vi "Shot Counter.vi"() -> ()   [LabVIEW 2013]
uses:
  <vilib>/Utility/file.llb/Write To Spreadsheet File (DBL).vi
  <vilib>/Utility/file.llb/Read From Spreadsheet File (I64).vi
  <vilib>/Utility/file.llb/Write To Spreadsheet File (I64).vi
  Globals/Useful Values.vi
panel:
  out "Time":i64
  out "Shots":i64
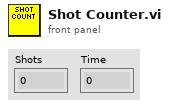
[diagram p1: front panel]
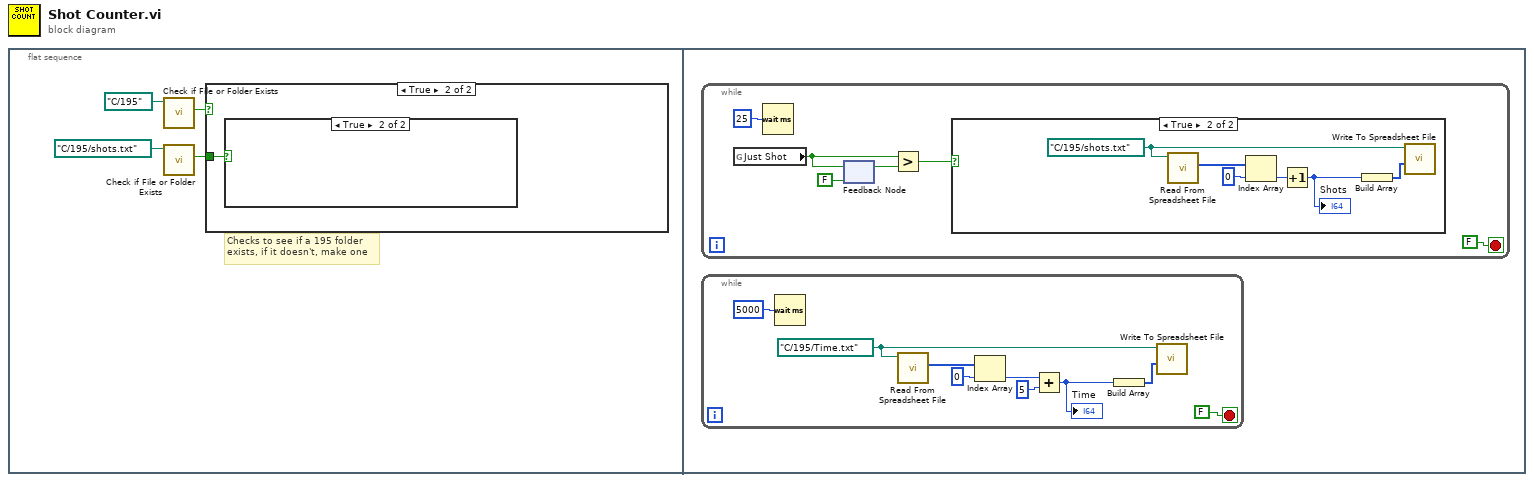
[diagram p0: block diagram]
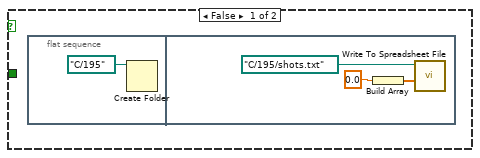
[diagram p2: hidden frame]
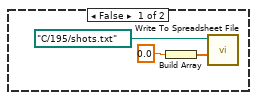
[diagram p3: hidden frame]
diagram:
  n1 = flat-sequence {
    frame #0 {
      # "Checks to see if a 195 folder\nexists, if it doesn't, make one"
      n2 = call <vilib>:"Check if File or Folder Exists.vi"("path"=path "C:/195") -> ("file or folder exists?"=w2:bool)  [unwired: 8 in, 2 out]
      n3 = call <vilib>:"Check if File or Folder Exists.vi"("path"=path "C:/195/shots.txt") -> ("file or folder exists?"=w1:bool)  [unwired: 8 in, 2 out]
      n4 = case shown="True" w2 {
        tunnel: w1 -> [_ w9]
        frame False {
          n5 = flat-sequence {
            frame #0 {
              n6 = Create Folder(path (use dialog)=path "C:/195") -> ()  [unwired: 2 in, 3 out]
            }
            frame #1 {
              n7 = Build Array(0.0 ("element")) -> (w7:dbl[])
              n8 = call-poly <vilib>:"Write To Spreadsheet File.vi"("1D data"=w7, "file path (dialog if empty)"=path "C:/195/shots.txt") -> ()  [unwired: 6 in, 1 out]
            }
          }
        }
        frame True {
          n9 = case shown="True" w9 {
            frame False {
              n10 = Build Array(0.0 ("element")) -> (w11:dbl[])
              n11 = call-poly <vilib>:"Write To Spreadsheet File.vi"("1D data"=w11, "file path (dialog if empty)"=path "C:/195/shots.txt") -> ()  [unwired: 6 in, 1 out]
            }
            frame True {
            }
          }
        }
      }
    }
    frame #1 {
      n12 = while {
        stop <- FALSE stop-if-true
        n13 = global read "Useful Values.vi" "Just Shot"() -> (w26:bool)
        n14 = Wait (ms)(milliseconds to wait=u32 25) -> ()  [unwired: 1 out]
        n15 = feedback #1(FALSE ("Just Shot")) -> (w25:bool)
        n16 = feedback-in #1(w26) -> ()
        n17 = Greater?(x=w26, y=w25) -> (0:w27:bool)
        n18 = case shown="True" w27 {
          frame False {
          }
          frame True {
            w33 = path "C:/195/shots.txt" ("path")
            n19 = call-poly <vilib>:"Read From Spreadsheet File.vi"("file path (dialog if empty)"=w33) -> ("first row"=w31:i64[])  [unwired: 6 in, 4 out]
            n20 = Index Array(array=w31, index=0) -> (element=w29:i64)
            n21 = Increment(x=w29) -> (x+1=w30:i64)
            "Shots" <- w30
            n22 = Build Array(w30) -> (w28:i64[])
            n23 = call-poly <vilib>:"Write To Spreadsheet File.vi"("1D data"=w28, "file path (dialog if empty)"=w33) -> ()  [unwired: 6 in, 1 out]
          }
        }
      }
      n24 = while {
        stop <- FALSE stop-if-true
        w14 = path "C:/195/Time.txt" ("path")
        n25 = Wait (ms)(milliseconds to wait=u32 5000) -> ()  [unwired: 1 out]
        n26 = call-poly <vilib>:"Read From Spreadsheet File.vi"("file path (dialog if empty)"=w14) -> ("first row"=w16:i64[])  [unwired: 6 in, 4 out]
        n27 = Index Array(array=w16, index=0) -> (element=w18:i64)
        n28 = Add(x=w18, y=i64 5 ("x")) -> (x+y=w17:i64)
        "Time" <- w17
        n29 = Build Array(w17) -> (w19:i64[])
        n30 = call-poly <vilib>:"Write To Spreadsheet File.vi"("1D data"=w19, "file path (dialog if empty)"=w14) -> ()  [unwired: 6 in, 1 out]
      }
    }
  }
